vi "Configure Offset and Limits (Spectrum Emission Mask - Relative And Absolute Limits).vi"(0 "VISA resource name":refnum<visa-resource-name>, 1 "Couple Relative Stop List":bool[](array[boolean])=[TRUE, TRUE, TRUE, TRUE, TRUE, TRUE], 2 "Manual Relative Stop List":dbl[](array[numeric])=[-30.0, -30.0, -30.0, -30.0, -30.0, -30.0] format="%#.6g", 3 "Couple Absolute Stop List":bool[](array[boolean])=[TRUE, TRUE, TRUE, TRUE, TRUE, TRUE], 5 "Device Mode (1: BTS)":i32(ring)=1 items=["BTS"=1, "MS"=2], 7 "Absolute Start List":dbl[](array[numeric])=[-14.0, -14.0, -14.0, -14.0, -14.0, -14.0] format="%#.6g", 9 "Manual Absolute Stop List":dbl[](array[numeric])=[-14.0, -14.0, -14.0, -14.0, -14.0, -14.0] format="%#.6g", 11 "error in (no error)":errorcluster, 12 "Relative Start List":dbl[](array[numeric])=[-30.0, -30.0, -30.0, -30.0, -30.0, -30.0] format="%#.6g", 13 "Fail Mask List":i32[](array[ring])=[0, 0, 0, 0, 0, 0] items=["Absolute", "Absolute And Relative", "Absolute Or Relative", "Relative"]) -> (4 "VISA resource name out":refnum<visa-resource-name>, 15 "error out":errorcluster)   [LabVIEW 2018, in "Agilent MXA Series.lvlib"]
doc: "Configures the Absolute and Relative Limit settings under the offsets and limits for Spectrum Emission Mask measurement type."
uses:
  Agilent MXA Series.lvlib
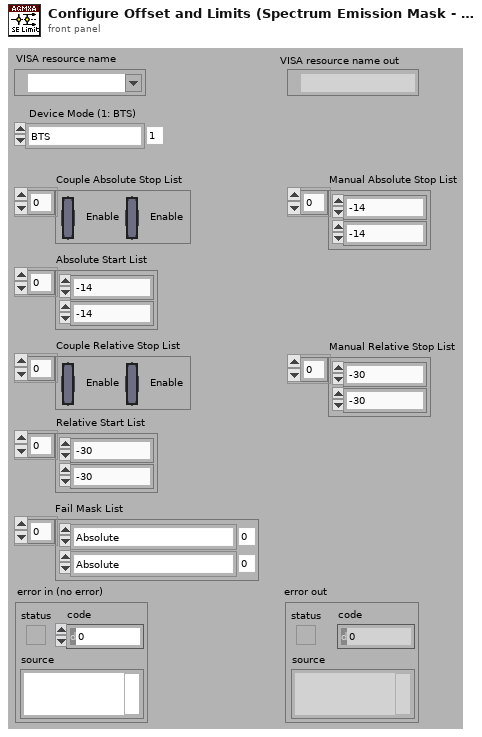
[diagram p1: front panel]
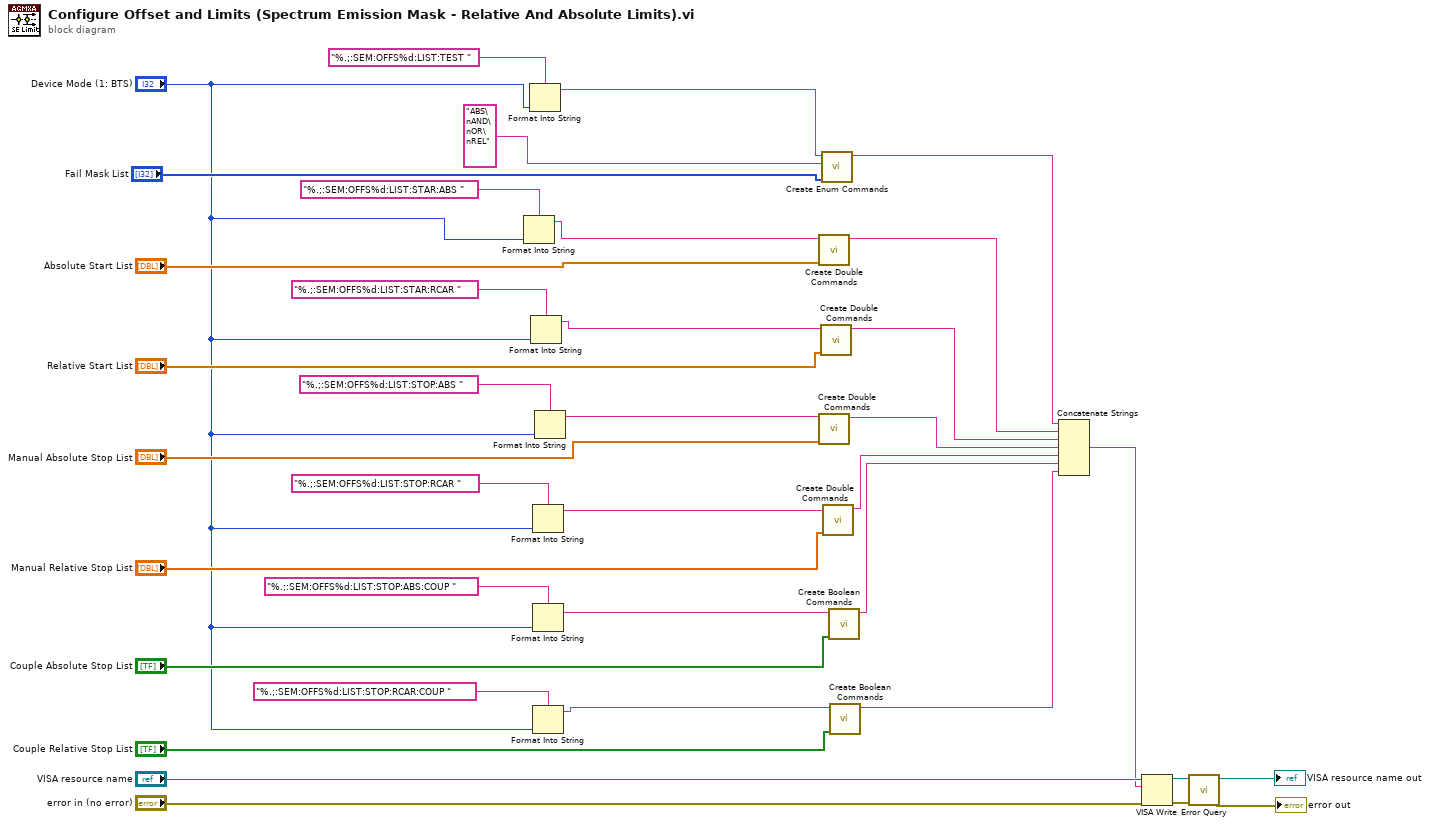
[diagram p0: block diagram]
diagram:
  n1 = Format Into String(format string="%.;:SEM:OFFS%d:LIST:STAR:ABS ", "Device Mode (1: BTS)") -> (resulting string=w35:string)  [unwired: 2 in, 1 out]
  n2 = Format Into String(format string="%.;:SEM:OFFS%d:LIST:TEST ", "Device Mode (1: BTS)") -> (resulting string=w5:string)  [unwired: 2 in, 1 out]
  n3 = Format Into String(format string="%.;:SEM:OFFS%d:LIST:STAR:RCAR ", "Device Mode (1: BTS)") -> (resulting string=w32:string)  [unwired: 2 in, 1 out]
  n4 = Format Into String(format string="%.;:SEM:OFFS%d:LIST:STOP:RCAR ", "Device Mode (1: BTS)") -> (resulting string=w26:string)  [unwired: 2 in, 1 out]
  n5 = Format Into String(format string="%.;:SEM:OFFS%d:LIST:STOP:ABS:COUP ", "Device Mode (1: BTS)") -> (resulting string=w23:string)  [unwired: 2 in, 1 out]
  n6 = Format Into String(format string="%.;:SEM:OFFS%d:LIST:STOP:RCAR:COUP ", "Device Mode (1: BTS)") -> (resulting string=w20:string)  [unwired: 2 in, 1 out]
  n7 = Format Into String(format string="%.;:SEM:OFFS%d:LIST:STOP:ABS ", "Device Mode (1: BTS)") -> (resulting string=w29:string)  [unwired: 2 in, 1 out]
  n8 = call "Create Double Commands.vi"("Double Values"="Absolute Start List", "Commands"=w35) -> ("Result"=w12:string)  [unwired: 9 in]
  n9 = call "Create Double Commands.vi"("Double Values"="Manual Absolute Stop List", "Commands"=w29) -> ("Result"=w10:string)  [unwired: 9 in]
  n10 = call "Create Double Commands.vi"("Double Values"="Relative Start List", "Commands"=w32) -> ("Result"=w11:string)  [unwired: 9 in]
  n11 = call "Create Enum Commands.vi"("Enum Values"="Fail Mask List", "Multi-line Text"="ABS\nAND\nOR\nREL" ("multi-line string"), "Commands"=w5) -> ("Result"=w2:string)  [unwired: 8 in]
  n12 = call "Create Double Commands.vi"("Double Values"="Manual Relative Stop List", "Commands"=w26) -> ("Result"=w9:string)  [unwired: 9 in]
  n13 = call "Create Boolean Commands.vi"("Boolean States"="Couple Absolute Stop List", "Command"=w23) -> ("Result String"=w8:string)  [unwired: 9 in]
  n14 = call "Create Boolean Commands.vi"("Boolean States"="Couple Relative Stop List", "Command"=w20) -> ("Result String"=w7:string)  [unwired: 9 in]
  n15 = Concatenate Strings(w2, w12, w11, w10, w9, w8, w7) -> (w6:string)
  n16 = VISA Write(VISA resource name="VISA resource name", write buffer=w6, error in (no error)="error in (no error)") -> (VISA resource name out=w17:refnum<visa-resource-name>, error out=w18:errorcluster)  [unwired: 1 out]
  n17 = call "Error Query.vi"("error in (no error)"=w18, "VISA resource name"=w17) -> ("error out"=→"error out":errorcluster, "VISA resource name out"=→"VISA resource name out":refnum<visa-resource-name>)  [unwired: 6 in, 2 out]
